vi "Connect Error Wires in Reset Case.vi"(0 "case sel refnum in":refnum<vi>, 11 "error in":errorcluster) -> (4 "case sel refnum out":refnum<vi>, 15 "error out":errorcluster)   [LabVIEW 2021, in "Converter.lvlib"]
uses:
  Converter.lvlib
  Converter Reusables/Converter Reusables.lvlib
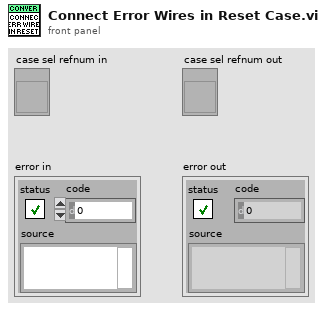
[diagram p1: front panel]
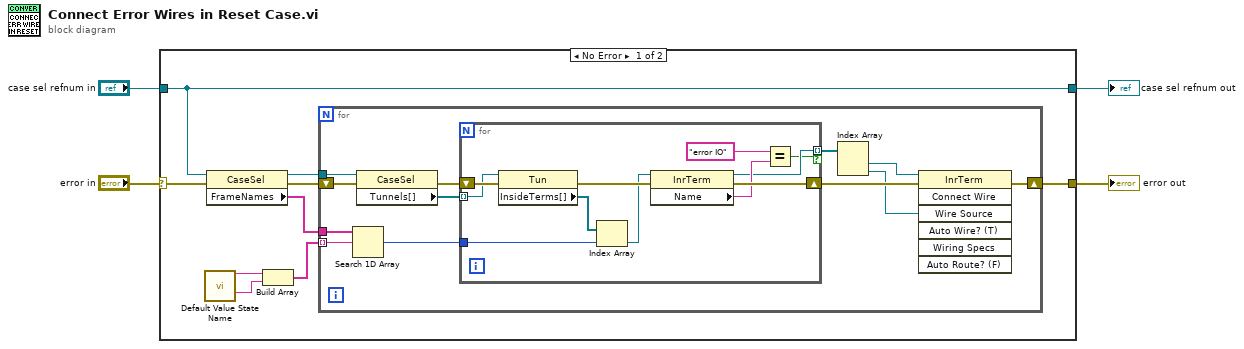
[diagram p0: block diagram]
diagram:
  n1 = case shown="No Error" "error in" {
    selector: "error in" -> [w12 w38]
    tunnel: [w9 w38] -> w4
    tunnel: "case sel refnum in" -> [w8 w37]
    tunnel: [w8 w37] -> w1
    frame No Error {
      n2 = call "Default Value State Name.vi"() -> ("set default value state"=w7:string, "load values"=w6:string)  [unwired: 12 in, 2 out]
      n3 = property class="CaseSel"(reference=w8, error in=w12) -> (reference out=w13:refnum<vi>, error out=w10:errorcluster, "FrameNames"=w11:string[])
      n4 = Build Array(w7, w6) -> (w5:string[])
      n5 = for {
        tunnel: w13 -> [w25]
        tunnel: w11 -> [w24]
        tunnel: w5 -> [w23] mode=indexing
        shift-right: [w19] -> w9
        shift-left: w10 -> [w22]
        n6 = Search 1D Array(1D array=w24, element=w23) -> (index of element=w17:i32)  [unwired: 1 in]
        n7 = property class="CaseSel"(reference=w25, error in=w22) -> (error out=w21:errorcluster, "Tunnels[]"=w18:refnum<vi>[])  [unwired: 1 out]
        n8 = for {
          shift-right: [w34] -> w20
          shift-left: w21 -> [w36]
          tunnel: w18 -> [w31] mode=indexing
          tunnel: w17 -> [w30]
          tunnel: [w28] -> w16 mode=indexing if=w27
          n9 = property class="Tun"(reference=w31, error in=w36) -> (error out=w35:errorcluster, "InsideTerms[]"=w32:refnum<vi>[])  [unwired: 1 out]
          n10 = Index Array(array=w32, index=w30) -> (element=w29:refnum<vi>)
          n11 = property class="InrTerm"(reference=w29, error in=w35) -> (reference out=w28:refnum<vi>, error out=w34:errorcluster, "Name"=w33:string)
          n12 = Equal?(x="error IO" ("y"), y=w33) -> (x = y?=w27:bool)
        }
        n13 = Index Array(array=w16) -> (element #1=w15:refnum<vi>, element #2=w14:refnum<vi>)  [unwired: 2 in]
        n14 = invoke class="InrTerm" method="Connect Wire"(reference=w15, error in=w20, "Wire Source"=w14) -> (error out=w19:errorcluster)  [unwired: 4 in, 6 out]
      }
    }
    frame Error {
    }
  }
  "error out" <- w4
  "case sel refnum out" <- w1
